vi "thcd_format_data.vi"(7 "n_max":i32=7200, 8 "array_in":cluster{"time":dbl, "value":dbl}[](array[cluster]), 10 "value":dbl, 11 "time":dbl) -> (0 "array_out":cluster{"time":dbl, "value":dbl}[](array[cluster]), 2 "cluster_out":cluster{cluster{"time":dbl, "value":dbl}[]})   [LabVIEW 2019]
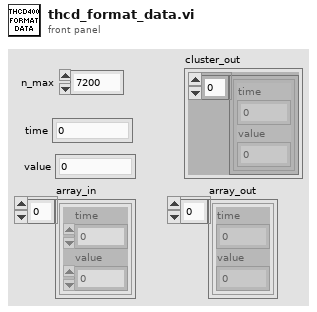
[diagram p1: front panel]
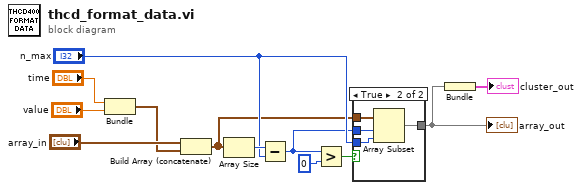
[diagram p0: block diagram]
diagram:
  n1 = Bundle("time"="time", "value"="value") -> (w3:cluster{"time":dbl, "value":dbl})  [unwired: 1 in]
  n2 = Build Array (concatenate) ("Sensor 1")("array_in", w3) -> (w5:cluster{"time":dbl, "value":dbl}[])
  n3 = Array Size(array=w5) -> (size(s)=w11:i32)
  n4 = Subtract(x=w11, y="n_max") -> (x-y=w9:i32)
  n5 = Greater?(x=w9, y=0) -> (0:w7:bool)
  n6 = case shown="True" w7 {
    tunnel: [w13 w17] -> w2
    tunnel: w5 -> [w13 w16]
    tunnel: "n_max" -> [_ w15]
    tunnel: w9 -> [_ w14]
    frame False {
    }
    frame True {
      n7 = Array Subset(array=w16, index=w14, length=w15) -> (w17:cluster{"time":dbl, "value":dbl}[])
    }
  }
  "array_out" <- w2
  n8 = Bundle(w2) -> (→"cluster_out":cluster{cluster{"time":dbl, "value":dbl}[]})  [unwired: 1 in]
